vi "FindDaysBackMin.vi"(10 "Cluster":cluster{i32[], timestamp[]}) -> (0 "Plot":T1(graph)=[{"Days"=[timestamp(3662524800 s since 1904-01-01), timestamp(3662611200 s since 1904-01-01), timestamp(3662697600 s since 1904-01-01), timestamp(3662784000 s since 1904-01-01), timestamp(3662870400 s since 1904-01-01), timestamp(3662956800 s since 1904-01-01), timestamp(3663043200 s since 1904-01-01), timestamp(3663129600 s since 1904-01-01), timestamp(3663216000 s since 1904-01-01), timestamp(3663302400 s since 1904-01-01), timestamp(3663388800 s since 1904-01-01), timestamp(3663475200 s since 1904-01-01), timestamp(3663561600 s since 1904-01-01), timestamp(3663648000 s since 1904-01-01), timestamp(3663734400 s since 1904-01-01), timestamp(3663820800 s since 1904-01-01), timestamp(3663907200 s since 1904-01-01), timestamp(3663993600 s since 1904-01-01), timestamp(3664080000 s since 1904-01-01), timestamp(3664166400 s since 1904-01-01), timestamp(3664252800 s since 1904-01-01), timestamp(3664339200 s since 1904-01-01), timestamp(3664425600 s since 1904-01-01), timestamp(3664512000 s since 1904-01-01), timestamp(3664598400 s since 1904-01-01), timestamp(3664684800 s since 1904-01-01), timestamp(3664771200 s since 1904-01-01), timestamp(3664857600 s since 1904-01-01), timestamp(3664944000 s since 1904-01-01), timestamp(3665030400 s since 1904-01-01), timestamp(3665116800 s since 1904-01-01), timestamp(3665203200 s since 1904-01-01), timestamp(3665289600 s since 1904-01-01), timestamp(3665376000 s since 1904-01-01), timestamp(3665462400 s since 1904-01-01), timestamp(3665548800 s since 1904-01-01), timestamp(3665635200 s since 1904-01-01), timestamp(3665721600 s since 1904-01-01), timestamp(3665808000 s since 1904-01-01), timestamp(3665894400 s since 1904-01-01), timestamp(3665980800 s since 1904-01-01), timestamp(3666067200 s since 1904-01-01), timestamp(3666153600 s since 1904-01-01), timestamp(3666240000 s since 1904-01-01), timestamp(3666326400 s since 1904-01-01), timestamp(3666412800 s since 1904-01-01), timestamp(3666499200 s since 1904-01-01), timestamp(3666585600 s since 1904-01-01), timestamp(3666672000 s since 1904-01-01), timestamp(3666758400 s since 1904-01-01), timestamp(3666844800 s since 1904-01-01), timestamp(3666931200 s since 1904-01-01), timestamp(3667017600 s since 1904-01-01), timestamp(3667104000 s since 1904-01-01), timestamp(3667190400 s since 1904-01-01), timestamp(3667276800 s since 1904-01-01), timestamp(3667363200 s since 1904-01-01), timestamp(3667449600 s since 1904-01-01), timestamp(3667536000 s since 1904-01-01), timestamp(3667622400 s since 1904-01-01), timestamp(3667708800 s since 1904-01-01), timestamp(3667795200 s since 1904-01-01), timestamp(3667881600 s since 1904-01-01), timestamp(3667968000 s since 1904-01-01), timestamp(3668054400 s since 1904-01-01), timestamp(3668140800 s since 1904-01-01), timestamp(3668227200 s since 1904-01-01), timestamp(3668313600 s since 1904-01-01), timestamp(3668400000 s since 1904-01-01), timestamp(3668486400 s since 1904-01-01), timestamp(3668572800 s since 1904-01-01), timestamp(3668659200 s since 1904-01-01), timestamp(3668745600 s since 1904-01-01), timestamp(3668832000 s since 1904-01-01)], "ConfirmedCases"=[0.0, 0.0, 0.0, 0.0, 0.0, 0.0, 0.0, 0.0, 0.0, 0.0, 0.0, 0.0, 0.0, 0.0, 0.0, 0.0, 0.0, 0.0, 0.0, 0.0, 0.0, 0.0, 0.0, 0.0, 0.0, 0.0, 0.0, 0.0, 0.0, 0.0, 0.0, 0.0, 0.0, 0.0, 0.0, 0.0, 0.0, 0.0, 0.0, 0.0, 0.0, 0.0, 1.0, 1.0, 1.0, 1.0, 1.0, 2.0, 3.0, 4.0, 4.0, 4.0, 4.0, 6.0, 11.0, 14.0, 17.0, 19.0, 24.0, 29.0, 33.0, 40.0, 52.0, 67.0, 83.0, 100.0, 121.0, 132.0, 149.0, 182.0, 212.0, 243.0, 282.0, 321.0]}, {"Days"=[timestamp(3668313600 s since 1904-01-01), timestamp(3668400000 s since 1904-01-01), timestamp(3668486400 s since 1904-01-01), timestamp(3668572800 s since 1904-01-01), timestamp(3668659200 s since 1904-01-01), timestamp(3668745600 s since 1904-01-01), timestamp(3668832000 s since 1904-01-01)], "ConfirmedCases"=[132.01823524302534, 153.55263572024907, 178.59966006386384, 207.73227646213113, 241.6169138771523, 281.0287070731711, 326.8692283660796]}, {"Days"=[timestamp(3668313600 s since 1904-01-01), timestamp(3668400000 s since 1904-01-01), timestamp(3668486400 s since 1904-01-01), timestamp(3668572800 s since 1904-01-01), timestamp(3668659200 s since 1904-01-01), timestamp(3668745600 s since 1904-01-01), timestamp(3668832000 s since 1904-01-01)], "ConfirmedCases"=[140.59609548662908, 162.8828644131387, 188.9766356577397, 219.6124606618654, 255.65531024069676, 298.10468948116306, 348.1074955925532]}, {"Days"=[timestamp(3668313600 s since 1904-01-01), timestamp(3668400000 s since 1904-01-01), timestamp(3668486400 s since 1904-01-01), timestamp(3668572800 s since 1904-01-01), timestamp(3668659200 s since 1904-01-01), timestamp(3668745600 s since 1904-01-01), timestamp(3668832000 s since 1904-01-01)], "ConfirmedCases"=[123.96371589380509, 144.75685960943596, 168.7924989452066, 196.49476425010758, 228.34938580605382, 264.9308682016178, 306.9267217896756]}, {"Days"=[timestamp(3668313600 s since 1904-01-01), timestamp(3668400000 s since 1904-01-01), timestamp(3668486400 s since 1904-01-01), timestamp(3668572800 s since 1904-01-01), timestamp(3668659200 s since 1904-01-01), timestamp(3668745600 s since 1904-01-01), timestamp(3668832000 s since 1904-01-01)], "ConfirmedCases"=[140.59609548662908, 160.133980854025, 182.38694136848164, 207.73227646213113, 236.5997168457177, 269.47871060219524, 306.9267217896756]}, {"Days"=[timestamp(3668313600 s since 1904-01-01), timestamp(3668400000 s since 1904-01-01), timestamp(3668486400 s since 1904-01-01), timestamp(3668572800 s since 1904-01-01), timestamp(3668659200 s since 1904-01-01), timestamp(3668745600 s since 1904-01-01), timestamp(3668832000 s since 1904-01-01)], "ConfirmedCases"=[123.96371589380509, 147.24177723483396, 174.89102199747728, 207.73227646213113, 246.7405026929383, 293.0737423477007, 348.1074955925532]}], 1 "Index":i32, 2 "Error":dbl, 3 "Growth":dbl)   [LabVIEW 2017]
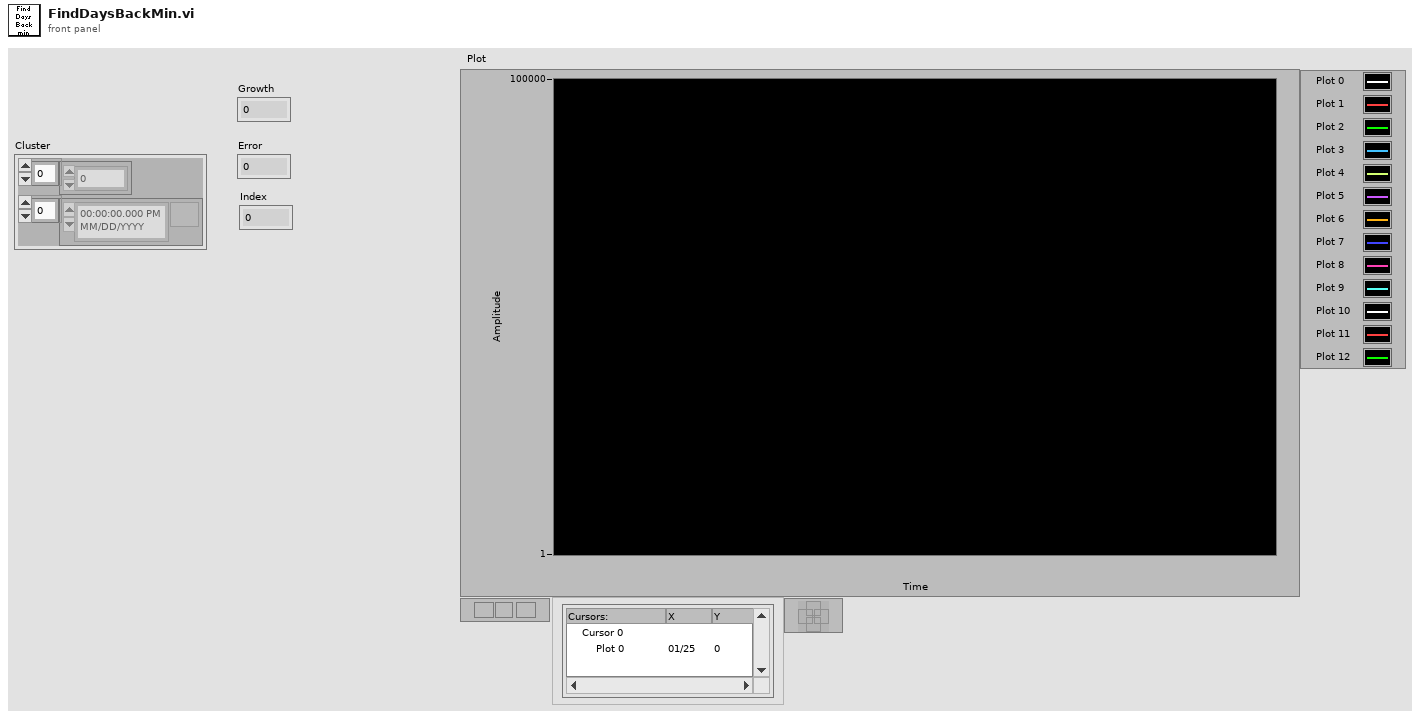
[diagram p1: front panel]
types:
  T1 = cluster{"Days":timestamp[], "ConfirmedCases":dbl[]}[]
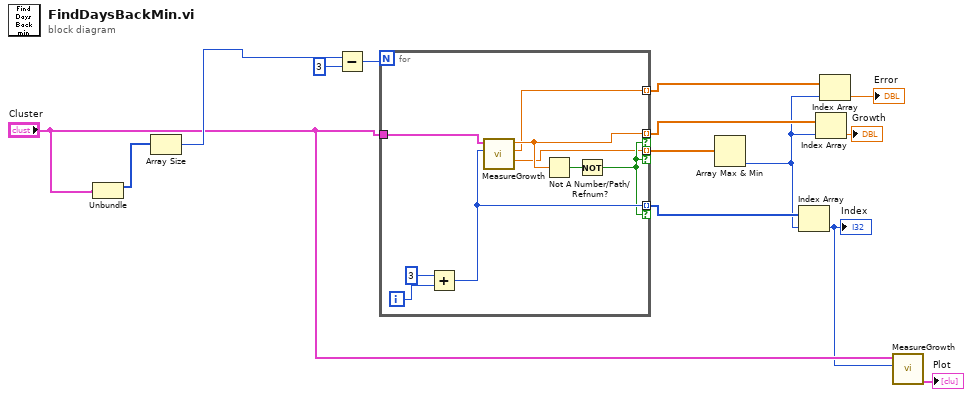
[diagram p0: block diagram]
diagram:
  n1 = Unbundle("Cluster") -> (w9:i32[])  [unwired: 1 out]
  n2 = Array Size(array=w9) -> (size(s)=w8:i32)
  n3 = Subtract(x=w8, y=3) -> (x-y=w11:i32)
  n4 = for {
    N: w11 -> [_]
    tunnel: "Cluster" -> [w17]
    tunnel: [w20] -> w13 mode=indexing if=w18
    tunnel: [w16] -> w12 mode=indexing if=w18
    tunnel: [w21] -> w7 mode=indexing if=w18
    tunnel: [w15] -> w6 mode=indexing
    i -> [w23]
    n5 = Add(x=3, y=w23) -> (x+y=w21:i32)
    n6 = call "MeasureGrowth.vi"("DaysBack"=w21, "Data"=w17) -> ("Interval"=w16:dbl, "PlusMinus"=w15:dbl, "Growth"=w20:dbl)  [unwired: 4 in, 3 out]
    n7 = Not A Number/Path/Refnum?(number/path/refnum=w20) -> (NaN/Path/Refnum?=w19:bool)
    n8 = Not(x=w19) -> (.not. x?=w18:bool)
  }
  n9 = Array Max & Min(array=w12) -> (min index (indices)=w5:i32)  [unwired: 3 out]
  n10 = Index Array(array=w7, index=w5) -> (element=w2:i32)
  "Index" <- w2
  n11 = Index Array(array=w13, index=w5) -> (element=→"Growth":dbl)
  n12 = Index Array(array=w6, index=w5) -> (element=→"Error":dbl)
  n13 = call "MeasureGrowth.vi"("DaysBack"=w2, "Data"="Cluster") -> ("Plot"=→"Plot":T1)  [unwired: 4 in, 5 out]
